vi "Apply CAN Configuration.vi"(7 "Restart (T)":bool=TRUE, 8 "error in (no error)":errorcluster, 10 "CAN Settings":T1={"Box ID"=1, "Publish Period (ms)"=5}, 11 "Ethernet in":refnum<class "ENET_BS1200.lvclass">) -> (0 "error out":errorcluster, 3 "Ethernet out":refnum<class "ENET_BS1200.lvclass">)   [LabVIEW 2021, in "BS120x Driver.lvlib" / "ENET_BS1200.lvclass"]
doc: "Sends the configuration updates to the Battery Simulator 1200. Changes will not be applied until after the unit is restarted. To apply multilple configuration settings in one set, set <b>Restart</b> to false on all Settings VIs except the last one.\n(c) 2019 Bloomy Controls, Inc. All rights reserved."
uses:
  ENET_BS1200.lvclass
  TypeDefs/CAN Settings.ctl
  <vilib>/WebDAVClient/Advanced/Get Buffer.vi
  <vilib>/WebDAVClient/Advanced/Put Buffer.vi
  ENET_BS1200.lvclass/ENET_BS1200.ctl
  <vilib>/WebDAVClient/NI_WebDAV.lvlib
  BS120x.lvclass
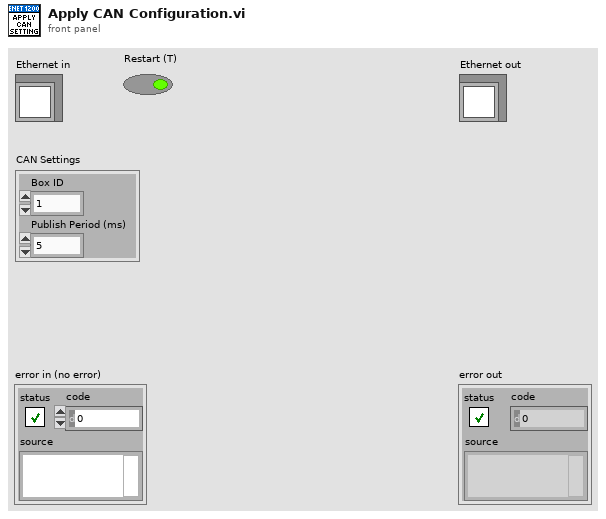
[diagram p1: front panel]
types:
  T1 = typedef "BS120x Driver.lvlib/BS120x.lvclass/CAN Settings.ctl" = cluster{"Box ID":i32, "Publish Period (ms)":i32}
  T2 = typedef "NI_WebDAV.lvlib/SessionHandle.ctl" = refnum<k1>
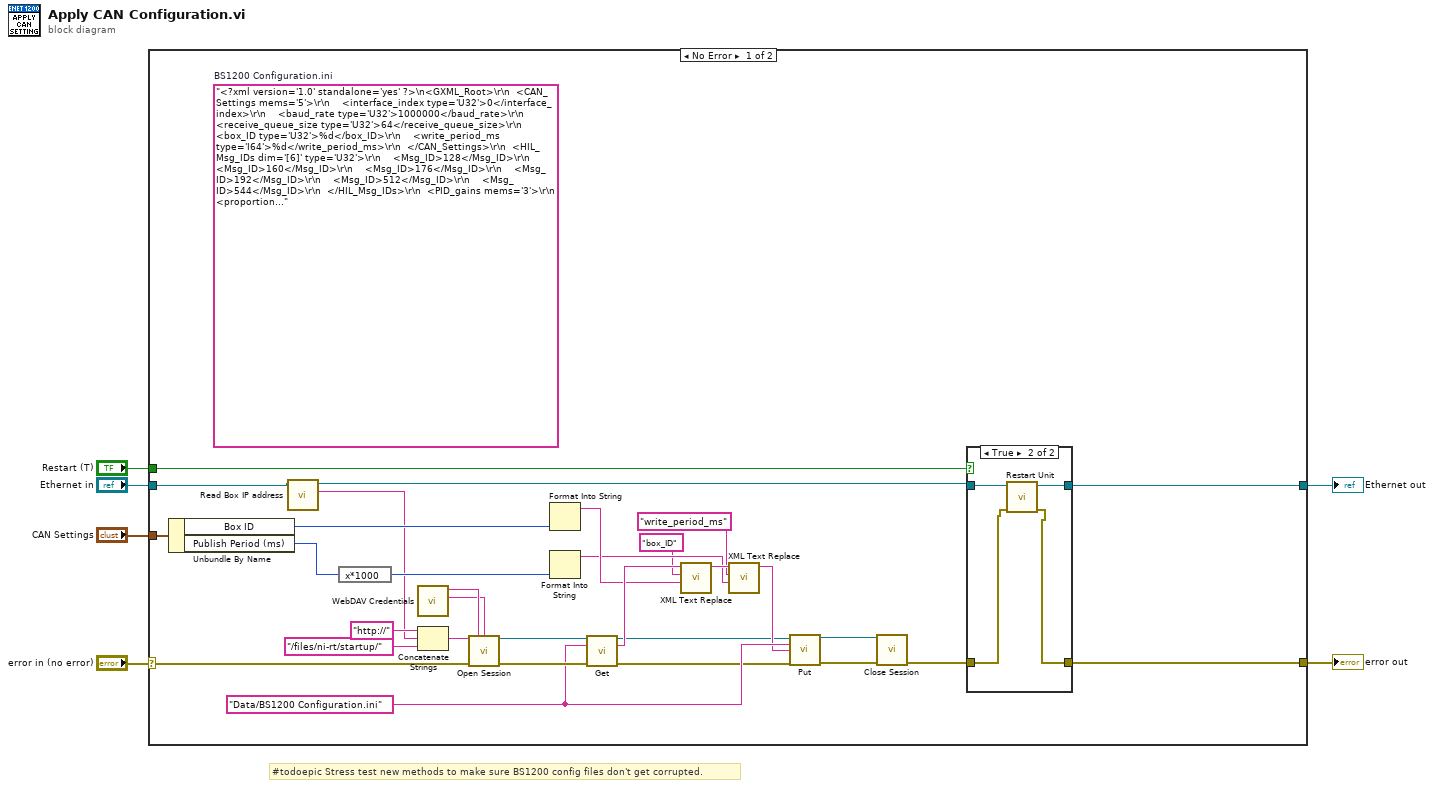
[diagram p0: block diagram]
diagram:
  # "#todoepic Stress test new methods to make sure BS1200 config files don't get corrupted."
  n1 = case shown="No Error" "error in (no error)" {
    selector: "error in (no error)" -> [w35 w45]
    tunnel: [w26 w45] -> w5
    tunnel: [w27 w44] -> w3
    tunnel: "Ethernet in" -> [w9 w44]
    tunnel: "CAN Settings" -> [w31 _]
    tunnel: "Restart (T)" -> [w25 _]
    frame No Error {
      (unwired) "<?xml version='1.0' standalone='yes' ?>\n<GXML_Root>\r\n  <CAN_Settings mems='5'>\r\n    <interface_index type='U32'>0</interface_index>\r\n    <baud_rate type='U32'>1000000</baud_rate>\r\n    <receive_queue_size type='U32'>64</receive_queue_size>\r\n    <box_ID type='U32'>%d</box_ID>\r\n    <write_period_ms type='I64'>%d</write_period_ms>\r\n  </CAN_Settings>\r\n  <HIL_Msg_IDs dim='[6]' type='U32'>\r\n    <Msg_ID>128</Msg_ID>\r\n    <Msg_ID>160</Msg_ID>\r\n    <Msg_ID>176</Msg_ID>\r\n    <Msg_ID>192</Msg_ID>\r\n    <Msg_ID>512</Msg_ID>\r\n    <Msg_ID>544</Msg_ID>\r\n  </HIL_Msg_IDs>\r\n  <PID_gains mems='3'>\r\n    <proportional_gain type='DBL'>0.3</proportional_gain>\r\n    <integral_gain type='DBL'>0.55</integral_gain>\r\n    <derivative_gain type='DBL'>0</derivative_gain>\r\n  </PID_gains>\r\n  <Enable_Cell_Inhibit type='Bool'>FALSE</Enable_Cell_Inhibit>\r\n</GXML_Root>"  # BS1200 Configuration.ini
      w19 = "Data/BS1200 Configuration.ini" ("string")
      n2 = Unbundle By Name(w31) -> ("Box ID"=w22:i32, "Publish Period (ms)"=w24:i32)
      n3 = call-dynamic "Read Box IP address.vi"("ENET_BS120x in"=w9) -> ("Box IP address"=w7:string, "ENET_BS120x out"=w8:refnum<class "ENET_BS1200.lvclass">)  [unwired: 8 in, 1 out]
      n4 = expression code="x*1000"(w24) -> (w21:i32)
      n5 = call "WebDAV Credentials.vi"() -> ("Password"=w33:string, "Username"=w34:string)  [unwired: 10 in]
      n6 = Concatenate Strings("http://" ("string"), w7, "/files/ni-rt/startup/" ("string")) -> (w32:string)
      n7 = call <vilib>:"Open Session.vi"("host uri prefix"=w32, "username"=w34, "password"=w33, "error in (no error)"=w35) -> ("session handle out"=w23:T2, "error out"=w20:errorcluster)  [unwired: 10 in]
      n8 = Format Into String(w22) -> (resulting string=w15:string)  [unwired: 3 in, 1 out]
      n9 = Format Into String(w21) -> (resulting string=w14:string)  [unwired: 3 in, 1 out]
      n10 = call-poly <vilib>:"Get.vi"("session handle"=w23, "relative uri"=w19, "error in (no error)"=w20) -> ("session handle out"=w10:T2, "data"=w18:string, "error out"=w11:errorcluster)  [unwired: 10 in]
      n11 = call "XML Text Replace.vi"("Text"=w15, "Tag"="box_ID", "XML in"=w18) -> ("XML out"=w16:string)  [unwired: 8 in]
      n12 = call "XML Text Replace.vi"("Text"=w14, "Tag"="write_period_ms", "XML in"=w16) -> ("XML out"=w17:string)  [unwired: 8 in]
      n13 = call-poly <vilib>:"Put.vi"("session handle"=w10, "relative uri"=w19, "data"=w17, "error in (no error)"=w11) -> ("session handle out"=w30:T2, "error out"=w29:errorcluster)  [unwired: 10 in]
      n14 = call <vilib>:"Close Session.vi"("session handle"=w30, "error in (no error)"=w29) -> ("error out"=w28:errorcluster)  [unwired: 13 in]
      n15 = case shown="True" w25 {
        tunnel: [w39 w40] -> w26
        tunnel: [w38 w41] -> w27
        tunnel: w28 -> [w39 w43]
        tunnel: w8 -> [w38 w42]
        frame False {
        }
        frame True {
          n16 = call-dynamic "Restart Unit.vi"("error in (no error)"=w43, "ENET in"=w42) -> ("error out"=w40:errorcluster, "ENET out"=w41:refnum<class "ENET_BS1200.lvclass">)  [unwired: 8 in]
        }
      }
    }
    frame Error {
    }
  }
  "error out" <- w5
  "Ethernet out" <- w3
